vi "PathPlanner_Auto_FromAutoFile.vi"(11 "FileName":string="Auto.auto") -> (0 "error out":errorcluster, 2 "Auto Command":T1, 4 "Full Filename":string)   [LabVIEW 2023]
uses:
  <vilib>/Rock Robotics/WPI/ThirdParty/MJansen/PathPlanner/TypeDef/PathPlannerCommandUtil.ctl
  <vilib>/Rock Robotics/WPI/ThirdParty/MJansen/PathPlanner/ENum/PathPlanner_CommandUtilType_ENUM.ctl
  <vilib>/Rock Robotics/WPI/ThirdParty/JAS_Junk/TrajLib/Conv_Deg_Radians.vi
  <vilib>/Rock Robotics/WPI/ThirdParty/JAS_Junk/TrajLib/Rotation2d_CreateAngle.vi
  <vilib>/Rock Robotics/WPI/ThirdParty/MJansen/PathPlanner/PathPlanner24.lvlib
  <vilib>/Rock Robotics/WPI/ThirdParty/JAS_Junk/TrajLib/TypeDef/TRANSLATION2D.ctl
  <vilib>/Rock Robotics/WPI/ThirdParty/JAS_Junk/TrajLib/Trajectory_Library.lvlib
  <vilib>/Rock Robotics/WPI/ThirdParty/JAS_Junk/TrajLib/TypeDef/ROTATION2D.ctl
  <vilib>/Rock Robotics/WPI/ThirdParty/JAS_Junk/TrajLib/TypeDef/POSE2D.ctl
panel:
  in  "command":T3
  in  "error in (no error)":errorcluster
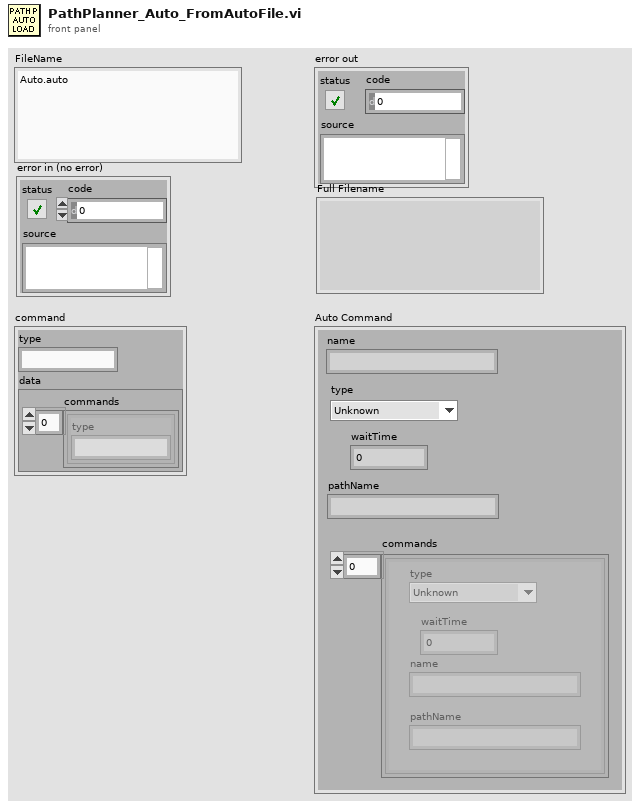
[diagram p1: front panel]
types:
  T1 = typedef "PathPlanner24.lvlib/PathPlannerCommandUtil.ctl" = cluster{"waitTime":dbl, "name":string, "pathName":string, "commands":cluster{"type":T2, "waitTime":dbl, "name":string, "pathName":string}[], "type":T2}
  T2 = typedef "PathPlanner24.lvlib/PathPlanner_CommandUtilType_ENUM.ctl" = enum16{"Unknown", "Wait", "Named", "Path", "Sequential", "Parallel", "Race", "Deadline"}
  T3 = cluster{"type":string, "data":cluster{"commands":cluster{"type":string}[]}}
  T4 = enum16{"open", "replace", "create", "open or create", "replace or create", "replace or create with confirmation"}
  T5 = cluster{"type":T2, "waitTime":dbl, "name":string, "pathName":string}
  T6 = typedef "Trajectory_Library.lvlib/POSE2D.ctl" = cluster{"TRANSLATION":T7, "ROTATION":T8}
  T7 = typedef "Trajectory_Library.lvlib/TRANSLATION2D.ctl" = cluster{"X":dbl, "Y":dbl}
  T8 = typedef "Trajectory_Library.lvlib/ROTATION2D.ctl" = cluster{"VALUE":dbl, "COS":dbl, "SIN":dbl}
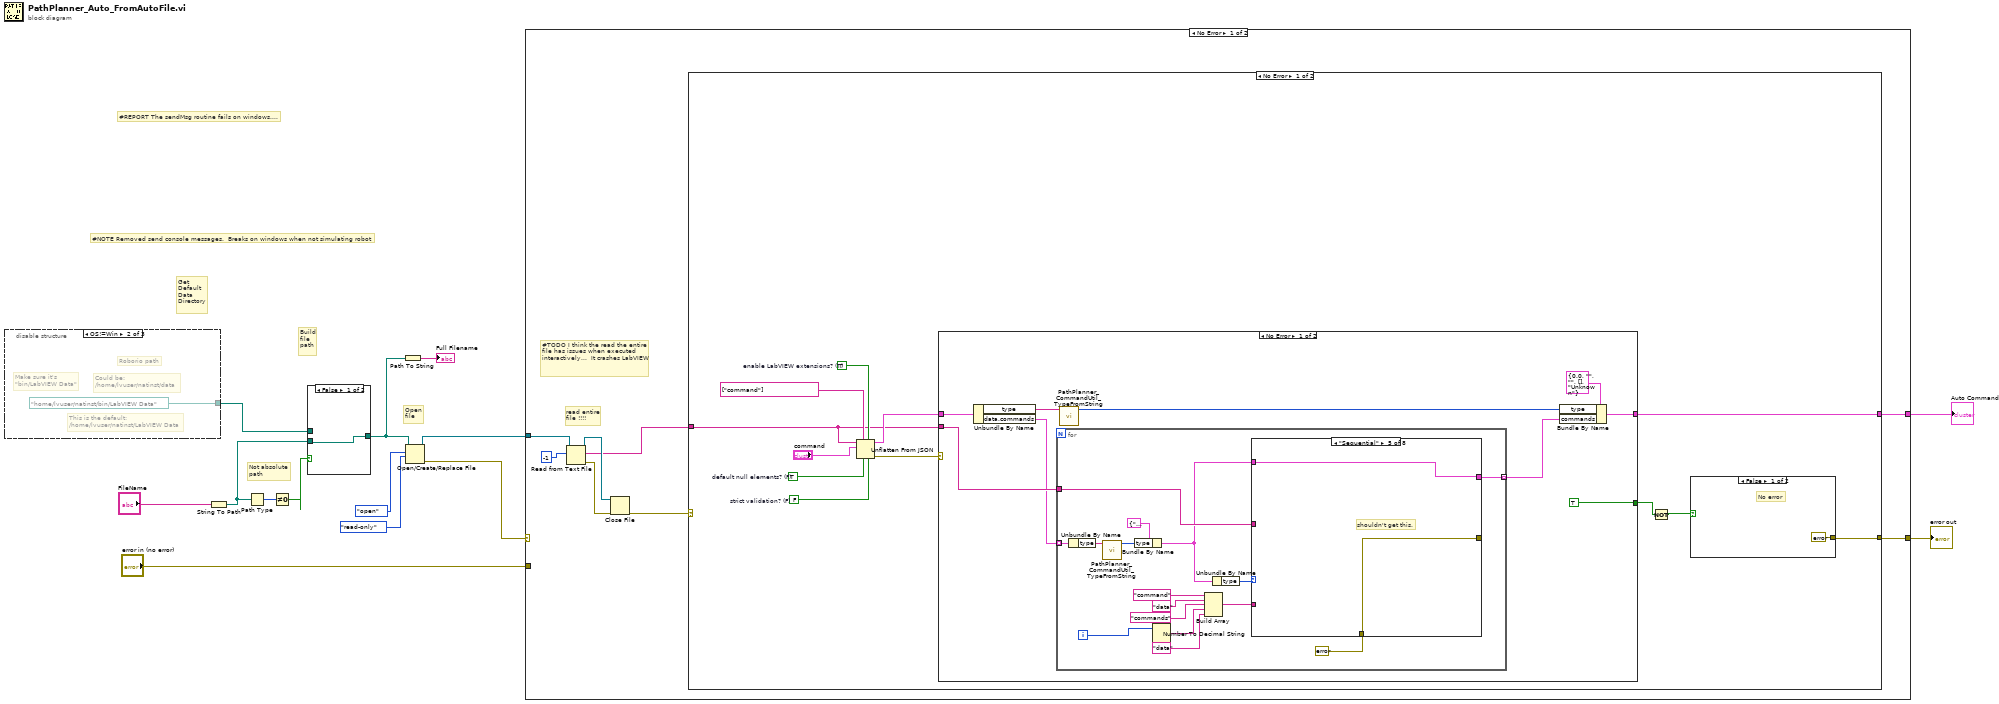
[diagram p0: block diagram]
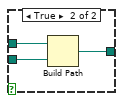
[diagram p2: hidden frame]
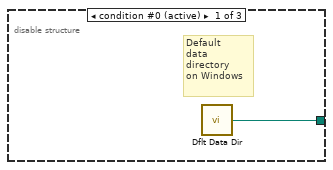
[diagram p3: hidden frame]
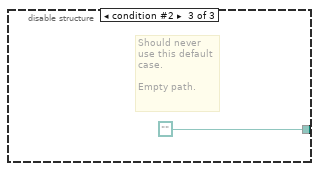
[diagram p4: hidden frame]
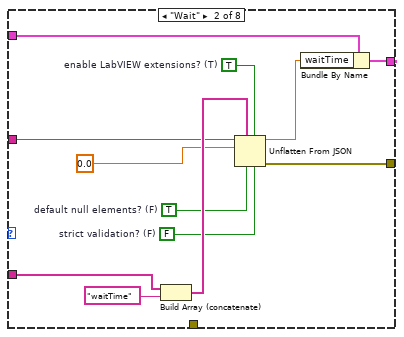
[diagram p6: hidden frame]
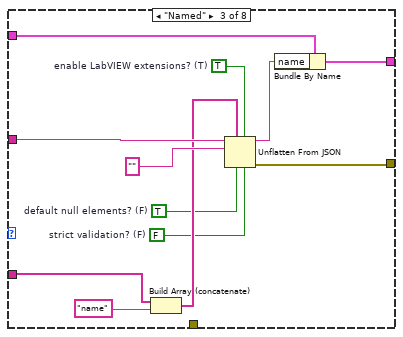
[diagram p7: hidden frame]
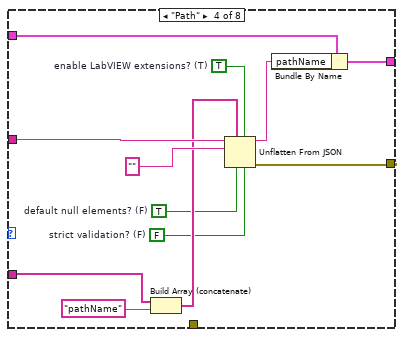
[diagram p8: hidden frame]
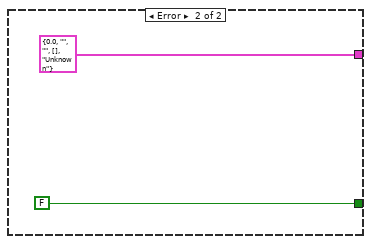
[diagram p12: hidden frame]
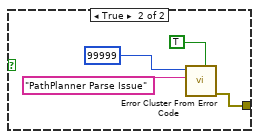
[diagram p13: hidden frame]
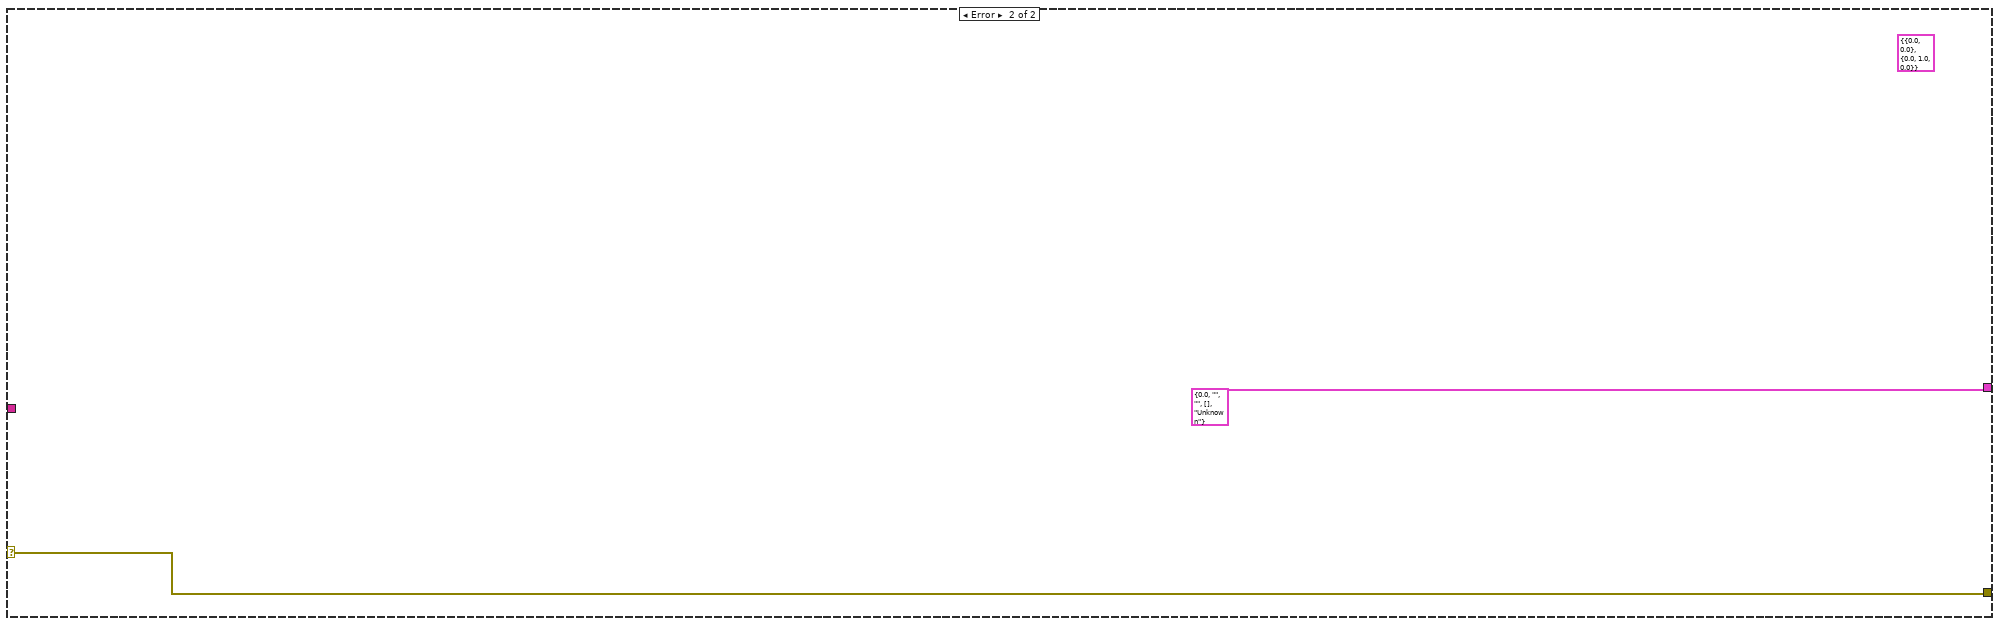
[diagram p14: hidden frame]
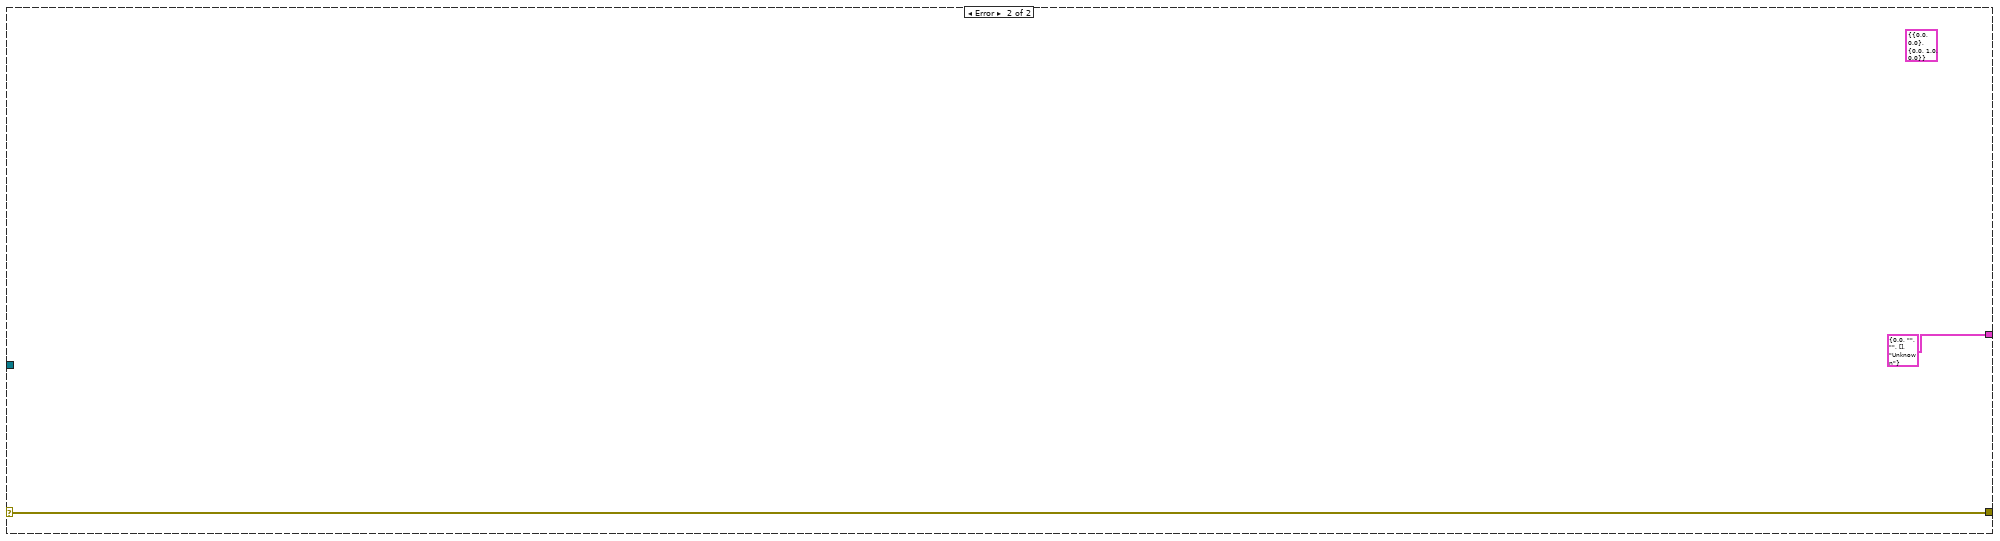
[diagram p15: hidden frame]
diagram:
  # "Not absolute\npath"
  # "#NOTE Removed send console messages.  Breaks on windows when not simulating robot"
  # "#REPORT The sendMsg routine fails on windows...."
  # "Get\nDefault\nData\nDirectory"
  # "Open\nfile"
  # "Build\nfile\npath"
  n1 = disable-structure shown="OS!=Win" {
    disable-tunnel: [w15 path "/home/lvuser/natinst/bin/LabVIEW Data" path ""] -> w11
    frame condition #0 (active) {
      # "Default\ndata\ndirectory\non Windows"
      n2 = call <vilib>:"Dflt Data Dir.vi"() -> ("App:Default Data Directory"=w15:path)
    }
    frame condition #1 {
      # "Make sure it's \n\"bin/LabVIEW Data\""
      # "This is the default:\n/home/lvuser/natinst/LabVIEW Data"
      # "Could be:\n/home/lvuser/natinst/data"
      # "Roborio path"
    }
    frame condition #2 {
      # "Should never\nuse this default\ncase.\n\nEmpty path."
    }
  }
  n3 = String To Path(string="FileName") -> (path=w10:path)
  n4 = Path Type(1:w10) -> (0:w9:i16)
  n5 = Not Equal To 0?(x=w9) -> (x != 0?=w8:bool)
  n6 = case shown="False" w8 {
    tunnel: [w18 w21] -> w5
    tunnel: w11 -> [_ w20]
    tunnel: w10 -> [w18 w19]
    frame False {
    }
    frame True {
      n7 = Build Path(base path=w20, name or relative path=w19) -> (appended path=w21:path)
    }
  }
  n8 = Path To String(path=w5) -> (string=→"Full Filename":string)
  n9 = Open/Create/Replace File(file path (use dialog)=w5, operation (0:open)=T4."open", access (0:read/write)=enum16{"read/write", "read-only", "write-only"}."read-only") -> (refnum out=w6:refnum<file>, error out=w12:errorcluster)  [unwired: 3 in, 1 out]
  n10 = case shown="No Error" w12 {
    selector: w12 -> [_ w123]
    tunnel: w6 -> [w28 _]
    tunnel: [w23 w123] -> w2
    tunnel: "error in (no error)" -> [_ _]
    tunnel: [w22 T1 {"waitTime"=0.0, "name"="", "pathName"="", "commands"=[], "type"=enum."Unknown"} ("Command")] -> w1
    frame No Error {
      # "#TODO I think the read the entire\nfile has issues when executed\ninteractively...  It crashes LabVIEW"
      # "read entire\nfile !!!!"
      n11 = Read from Text File(file (use dialog)=w28, count=-1) -> (refnum out=w27:refnum<file>, text=w26:string, error out=w25:errorcluster)  [unwired: 2 in, 1 out]
      n12 = Close File(refnum=w27, error in=w25) -> (error out=w24:errorcluster)  [unwired: 1 out]
      n13 = case shown="No Error" w24 {
        selector: w24 -> [_ w121]
        tunnel: w26 -> [w31 _]
        tunnel: [w41 w121] -> w23
        tunnel: [w32 T1 {"waitTime"=0.0, "name"="", "pathName"="", "commands"=[], "type"=enum."Unknown"} ("Command")] -> w22
        frame No Error {
          w37 = FALSE  # strict validation? (F)
          w38 = TRUE  # default null elements? (F)
          w39 = TRUE  # enable LabVIEW extensions? (T)
          n14 = Unflatten From JSON(path=string[] ["command"] ("path 2"), enable LabVIEW extensions? (T)=w39, JSON string=w31, type and defaults="command", default null elements? (F)=w38, strict validation? (F)=w37) -> (value=w36:T3, error out=w35:errorcluster)  [unwired: 1 in]
          n15 = case shown="No Error" w35 {
            tunnel: w36 -> [w50 _]
            tunnel: [TRUE FALSE] -> w33
            tunnel: [w42 T1 {"waitTime"=0.0, "name"="", "pathName"="", "commands"=[], "type"=enum."Unknown"} ("Command")] -> w32
            tunnel: w31 -> [w48 _]
            frame No Error {
              n16 = Unbundle By Name(w50) -> ("type"=w45:string, "data.commands"=w46:cluster{"type":string}[])
              n17 = for {
                tunnel: w46 -> [w66] mode=indexing
                tunnel: [w51] -> w43 mode=indexing
                tunnel: w48 -> [w54]
                i -> [w52]
                n18 = Unbundle By Name(w66) -> ("type"=w64:string)
                n19 = call <vilib>:"PathPlanner_CommandUtil_TypeFromString.vi"("Type string"=w64) -> ("Type"=w65:T2)  [unwired: 10 in]
                n20 = Bundle By Name(cluster=T5 {"type"=enum."Unknown", "waitTime"=0.0, "name"="", "pathName"=""} ("Command"), "type"=w65) -> (w53:T5)
                n21 = Number To Decimal String(number=w52) -> (decimal integer string=w58:string)  [unwired: 1 in]
                n22 = Build Array("command", "data", "commands", w58, "data") -> (w56:string[])
                n23 = Unbundle By Name(w53) -> ("type"=w62:T2)
                n24 = case shown="\"Sequential\"" w62 {
                  tunnel: w53 -> [w68 w73 w83 w95 w106 w108 w110 w112]
                  tunnel: [w68 w70 w84 w96 w106 w108 w110 w112] -> w51
                  tunnel: w56 -> [_ w74 w92 w104 _ _ _ _]
                  tunnel: w54 -> [_ w72 w90 w102 _ _ _ _]
                  tunnel: [w67 w69 w81 w93 w105 w107 w109 w111] -> _
                  tunnel: errorcluster {"status"=FALSE, "code"=0, "source"=""} ("error out") -> [w67 _ _ _ w105 w107 w109 w111]
                  frame "Unknown", Default {
                  }
                  frame "Wait" {
                    w76 = FALSE  # strict validation? (F)
                    w77 = TRUE  # default null elements? (F)
                    w78 = TRUE  # enable LabVIEW extensions? (T)
                    n25 = Build Array (concatenate)(w74, "waitTime") -> (w79:string[])
                    n26 = Unflatten From JSON(path=w79, enable LabVIEW extensions? (T)=w78, JSON string=w72, type and defaults=0.0, default null elements? (F)=w77, strict validation? (F)=w76) -> (value=w75:dbl, error out=w69:errorcluster)  [unwired: 1 in]
                    n27 = Bundle By Name(cluster=w73, "waitTime"=w75) -> (w70:T5)
                  }
                  frame "Named" {
                    w85 = FALSE  # strict validation? (F)
                    w86 = TRUE  # default null elements? (F)
                    w87 = TRUE  # enable LabVIEW extensions? (T)
                    n28 = Build Array (concatenate)(w92, "name") -> (w88:string[])
                    n29 = Unflatten From JSON(path=w88, enable LabVIEW extensions? (T)=w87, JSON string=w90, type and defaults="", default null elements? (F)=w86, strict validation? (F)=w85) -> (value=w82:string, error out=w81:errorcluster)  [unwired: 1 in]
                    n30 = Bundle By Name(cluster=w83, "name"=w82) -> (w84:T5)
                  }
                  frame "Path" {
                    w97 = FALSE  # strict validation? (F)
                    w98 = TRUE  # default null elements? (F)
                    w99 = TRUE  # enable LabVIEW extensions? (T)
                    n31 = Build Array (concatenate)(w104, "pathName") -> (w100:string[])
                    n32 = Unflatten From JSON(path=w100, enable LabVIEW extensions? (T)=w99, JSON string=w102, type and defaults="", default null elements? (F)=w98, strict validation? (F)=w97) -> (value=w94:string, error out=w93:errorcluster)  [unwired: 1 in]
                    n33 = Bundle By Name(cluster=w95, "pathName"=w94) -> (w96:T5)
                  }
                  frame "Sequential" {
                    # "shouldn't get this."
                  }
                  frame "Parallel" {
                    # "Shouldn't get this."
                  }
                  frame "Race" {
                    # "Shouldn't get this."
                  }
                  frame "Deadline" {
                    # "Shouldn't get this."
                  }
                }
              }
              n34 = call <vilib>:"PathPlanner_CommandUtil_TypeFromString.vi"("Type string"=w45) -> ("Type"=w44:T2)  [unwired: 10 in]
              n35 = Bundle By Name(cluster=T1 {"waitTime"=0.0, "name"="", "pathName"="", "commands"=[], "type"=enum."Unknown"} ("Command"), "type"=w44, "commands"=w43) -> (w42:T1)
            }
            frame Error {
            }
          }
          n36 = Not(x=w33) -> (.not. x?=w34:bool)
          n37 = case shown="False" w34 {
            tunnel: [errorcluster {"status"=FALSE, "code"=0, "source"=""} ("error out") w116] -> w41
            frame False {
              # "No error"
            }
            frame True {
              n38 = call <vilib>:"Error Cluster From Error Code.vi"("is warning? (False)"=TRUE, "error message (\"\")"="PathPlanner Parse Issue" ("error message (\"\")"), "error code (0)"=99999) -> ("error out"=w116:errorcluster)  [unwired: 6 in]
            }
          }
        }
        frame Error {
          (unwired) T6 {"TRANSLATION"={"X"=0.0, "Y"=0.0}, "ROTATION"={"VALUE"=0.0, "COS"=1.0, "SIN"=0.0}} ("POSE2D")
        }
      }
    }
    frame Error {
      (unwired) T6 {"TRANSLATION"={"X"=0.0, "Y"=0.0}, "ROTATION"={"VALUE"=0.0, "COS"=1.0, "SIN"=0.0}} ("POSE2D")
    }
  }
  "error out" <- w2
  "Auto Command" <- w1
